vi "fgv_Cool down setup.vi"(0 "Function":enum16{"Intialize", "Write", "Read", "Clear"}(ring), 5 "Cool-down time (s)":dbl caption="Cool-down time (sec)" min=0.0 max=60.0 step=0.001 format="%#.3fs", 9 "Enable cool-down time":bool, 11 "error in (no error)":errorcluster) -> (6 "Cool-down time (s)":dbl caption="Cool-down time (sec)" min=0.0 max=60.0 step=0.001 format="%#.3fs", 10 "Enable cool-down time":bool, 15 "error out":errorcluster)   [LabVIEW 2013]
panel:
  # "Sub-Routine"
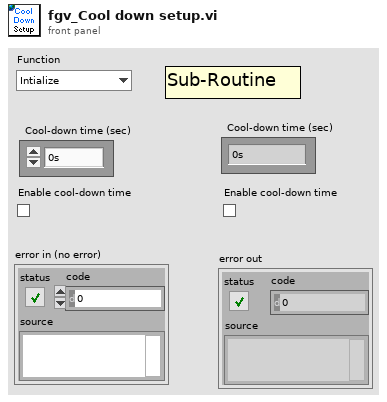
[diagram p1: front panel]
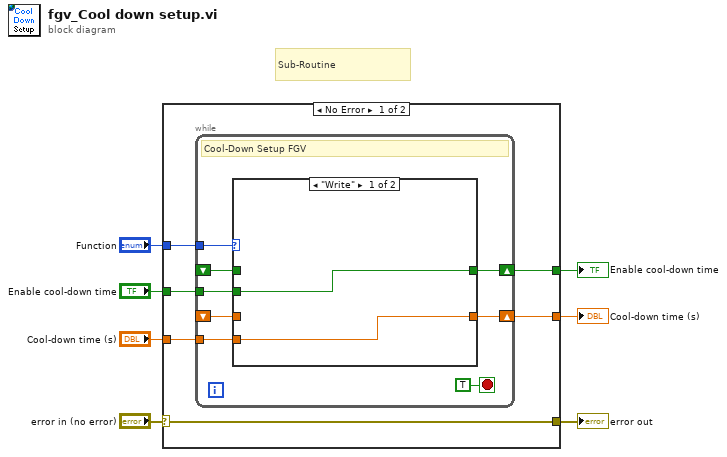
[diagram p0: block diagram]
diagram:
  # "Sub-Routine"
  n1 = case shown="No Error" "error in (no error)" {
    selector: "error in (no error)" -> [w8 w28]
    tunnel: [w8 w28] -> w5
    tunnel: "Function" -> [w13 _]
    tunnel: "Enable cool-down time" -> [w12 w27]
    tunnel: [w11 w27] -> w1
    tunnel: "Cool-down time (s)" -> [w10 w26]
    tunnel: [w9 w26] -> w2
    frame No Error {
      n2 = while {
        tunnel: w13 -> [w20]
        tunnel: w12 -> [w19]
        shift-right: [w18] -> w11
        shift-left: _ -> [w17]
        tunnel: w10 -> [w15]
        shift-right: [w16] -> w9
        shift-left: _ -> [w14]
        stop <- TRUE stop-if-true
        # "Cool-Down Setup FGV"
        n3 = case shown="\"Write\"" w20 {
          tunnel: [w23 w25] -> w18
          tunnel: w19 -> [w23 _]
          tunnel: w17 -> [_ w25]
          tunnel: [w22 w24] -> w16
          tunnel: w15 -> [w22 _]
          tunnel: w14 -> [_ w24]
          frame "Write" {
          }
          frame "Read", Default {
          }
        }
      }
    }
    frame Error {
    }
  }
  "error out" <- w5
  "Cool-down time (s)" <- w2
  "Enable cool-down time" <- w1
